vi "timming_array_to_digital_waveform.vi"(0 "resolution":i32=100, 1 "delay array":dbl[](array[numeric]) format="%#_6e", 2 "burst period":dbl, 3 "burst count":i32, 4 "Burst?":bool) -> (6 "digital waveform":digitalwaveform(waveform)={"t0"=timestamp(0 s since 1904-01-01), "dt"=0.0, "Y"={"transitions"=[], "data"=[]}, "error"={"status"=FALSE, "code"=37421928, "source"=""}})   [LabVIEW 2012]
doc: "takes the timing info recieved from the DG645 Delay generator and transforms it into a digital waveform graph.\nMakes sure, all timings are setup in reference to t0!"
panel:
  out "delta t":dbl
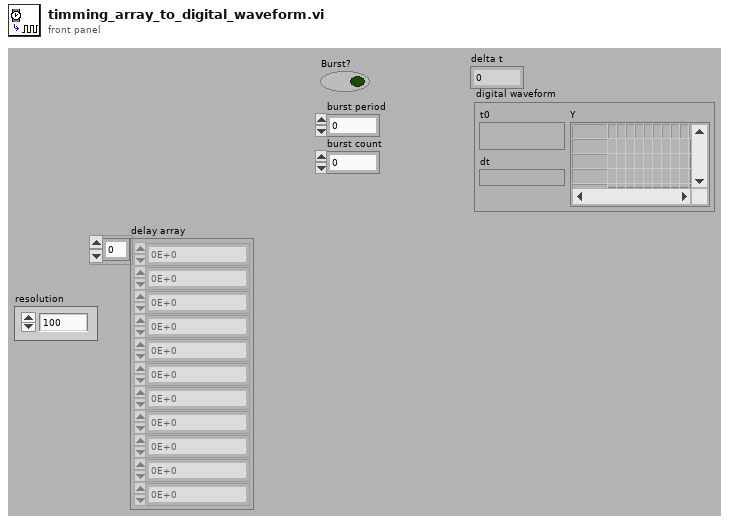
[diagram p1: front panel]
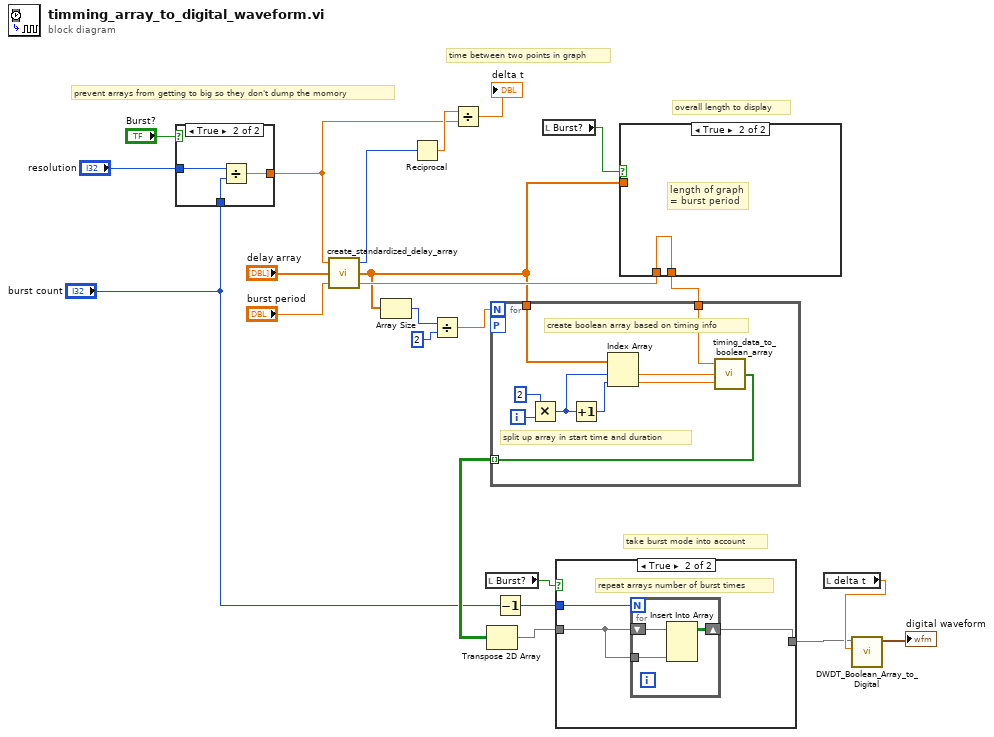
[diagram p0: block diagram]
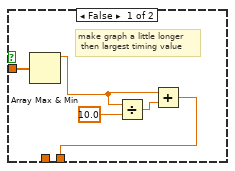
[diagram p4: hidden frame]
diagram:
  # "take burst mode into account"
  # "time between two points in graph"
  # "overall length to display"
  # "prevent arrays from getting to big so they don't dump the momory"
  n1 = case shown="True" "Burst?" {
    tunnel: [w24 w25] -> w12
    tunnel: "resolution" -> [w24 w27]
    tunnel: "burst count" -> [_ w26]
    frame False {
    }
    frame True {
      n2 = Divide(x=w27, y=w26) -> (x/y=w25:dbl)
    }
  }
  n3 = call "create_standardized_delay_array.vi"("burst period"="burst period", "delay array"="delay array", "resolution"=w12) -> ("corrected burst period"=w13:dbl, "standardize array"=w6:dbl[], "multiplier"=w19:i32)
  n4 = Array Size(array=w6) -> (size(s)=w2:i32)
  n5 = Reciprocal(x=w19) -> (1/x=w21:dbl)
  n6 = Divide(x=w2, y=2) -> (x/y=w1:dbl)
  n7 = Divide(x=w21, y=w12) -> (x/y=→"delta t":dbl)
  n8 = local read "Burst?"() -> (w18:bool)
  n9 = Decrement(x="burst count") -> (x-1=w17:i32)
  n10 = local read "Burst?"() -> (w9:bool)
  n11 = case shown="True" w9 {
    tunnel: [w31 w33] -> w22
    tunnel: w6 -> [w28 _]
    tunnel: w13 -> [_ w33]
    frame False {
      # "make graph a little longer\n then largest timing value"
      n12 = Array Max & Min(array=w28) -> (max value=w29:dbl)  [unwired: 3 out]
      n13 = Divide(x=w29, y=10.0) -> (x/y=w30:dbl)
      n14 = Add(x=w29, y=w30) -> (x+y=w31:dbl)
    }
    frame True {
      # "length of graph \n= burst period"
    }
  }
  n15 = for {
    N: w1 -> [_]
    tunnel: [w40] -> w23 mode=indexing
    tunnel: w22 -> [w39]
    tunnel: w6 -> [w34]
    workers-P: _ -> [_]
    i -> [w42]
    # "create boolean array based on timing info"
    # "split up array in start time and duration"
    n16 = Multiply(x=2, y=w42) -> (x*y=w35:i32)
    n17 = Increment(x=w35) -> (x+1=w38:i32)
    n18 = Index Array(array=w34, index #1=w35, index #2=w38) -> (element #1=w37:dbl, element #2=w36:dbl)
    n19 = call "timing_data_to_boolean_array.vi"("end time [s]"=w36, "start time [s]"=w37, "overall length [s]"=w39) -> ("boolean timing array"=w40:bool[])  [unwired: 1 in]
  }
  n20 = Transpose 2D Array(2D array=w23) -> (transposed array=w20:bool[][])
  n21 = case shown="True" w18 {
    tunnel: w20 -> [w43 w45]
    tunnel: [w43 w44] -> w10
    tunnel: w17 -> [_ w46]
    frame False {
    }
    frame True {
      # "repeat arrays number of burst times"
      n22 = for {
        N: w46 -> [_]
        shift-right: [w49] -> w44
        shift-left: w45 -> [w47]
        tunnel: w45 -> [w48]
        n23 = Insert Into Array(array=w47, new element=w48) -> (w49:bool[][])  [unwired: 2 in]
      }
    }
  }
  n24 = local read "delta t"() -> (w16:dbl)
  n25 = call "DWDT_Boolean_Array_to_Digital.vi"("delta t"=w16, "boolean array"=w10) -> ("digital waveform"=→"digital waveform":digitalwaveform)  [unwired: 8 in, 1 out]
